vi "Power Supply Enable All Out.vi"(10 "Enable":bool, 11 "ADALM2000 Handler":u32 caption="Instrument Handle Out") -> (3 "ADALM2000 Handler 2":u32 caption="Instrument Handle Out")   [LabVIEW 2015]
uses:
  libm2k_lv.dll
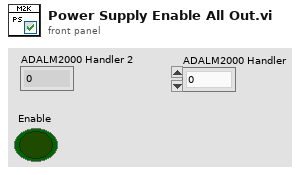
[diagram p1: front panel]
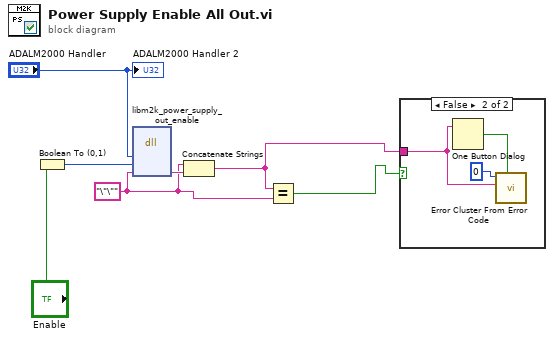
[diagram p0: block diagram]
diagram:
  w5 = "\"\""
  n1 = Boolean To (0,1)(Boolean="Enable") -> (0, 1=w3:i16)
  n2 = dll-call lib="libm2k_lv.*" fn="libm2k_power_supply_out_enable"("instance"="ADALM2000 Handler", "enable"=w3, "err"=w5) -> ("err"=w7:string)  [unwired: 6 in, 2 out]
  n3 = Concatenate Strings(w5, w7) -> (w1:string)
  n4 = Equal?(x=w1, y=w5) -> (x = y?=w2:bool)
  n5 = case shown="False" w2 {
    tunnel: w1 -> [_ w8]
    frame True {
    }
    frame False {
      n6 = One Button Dialog(message=w8) -> (true=w10:bool)  [unwired: 1 in]
      n7 = call <vilib>:"Error Cluster From Error Code.vi"("show call chain? (False)"=w10, "error message (\"\")"=w8, "error code (0)"=0) -> ()  [unwired: 6 in, 1 out]
    }
  }
  "ADALM2000 Handler 2" <- "ADALM2000 Handler"
